vi "Buffer VI Path by Type.vi"(10 "Packed Repeated":bool, 11 "Proto Type":T1) -> (2 "Decode":path, 3 "Encode":path)   [LabVIEW 2024, in "LV-Proto.lvlib"]
uses:
  LV-Proto.lvlib
  Proto Type.ctl
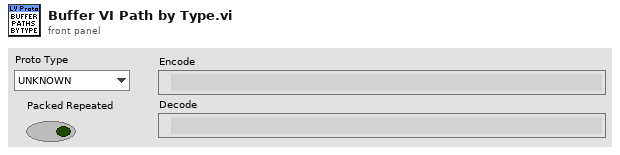
[diagram p1: front panel]
types:
  T1 = typedef "LV-Proto.lvlib/Proto Type.ctl" = enum16{"UNKNOWN", "double", "float", "int32", "int64", "uint32", "uint64", "sint32", "sint64", "fixed32", "fixed64", "sfixed32", "sfixed64", "bool", "string", "bytes", "enum", "map", "message"}
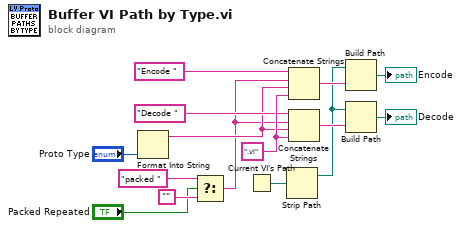
[diagram p0: block diagram]
diagram:
  w13 = ".vi" ("string")
  n1 = Format Into String("Proto Type") -> (resulting string=w10:string)  [unwired: 3 in, 1 out]
  n2 = Select(t="packed ", s="Packed Repeated", f="") -> (s? t:f=w1:string)
  n3 = Current VI's Path() -> (path=w15:path)
  n4 = Strip Path(path=w15) -> (stripped path=w7:path)  [unwired: 1 out]
  n5 = Concatenate Strings("Encode ", w1, w10, w13) -> (w9:string)
  n6 = Concatenate Strings("Decode ", w1, w10, w13) -> (w8:string)
  n7 = Build Path(base path=w7, name or relative path=w9) -> (appended path=→"Encode":path)
  n8 = Build Path(base path=w7, name or relative path=w8) -> (appended path=→"Decode":path)
